vi "GEMV_Benchmark(lv_gpu).vi"() -> ()   [LabVIEW 2020]
doc: "Solves the heat equation in a two-dimensional area using a Finite Element Method."
uses:
  <vilib>/addons/lvgpu/lvcuda/CUDA SGL Device Ptr/Download 2D Data.vi
  <vilib>/addons/lvgpu/lvcublas/SGEMM (aAB+bC).vi
  <vilib>/addons/lvgpu/lvcuda/CUDA SGL Device Ptr/Upload 1D Data.vi
  <vilib>/addons/lvgpu/lvcuda.lvlib
  <vilib>/addons/lvgpu/lvcublas.lvlib
  subVIs/Heat Equation Solver.lvlib
  <vilib>/addons/lvgpu/lvcuda/CUDA SGL Device Ptr/CUDA SGL Device Ptr.lvclass
  <vilib>/ptbypt/NI_PtbyPt.lvlib
panel:
  out "Heat Map":sgl[](array[numeric])
  out "Execution Time Graph":dbl(graph)
  out "Error Status":errorcluster
  out "time":dbl[unit] format="%#_4p"
  in  "stop":bool
  # "GEMV based on NI's GPU Toolkit"
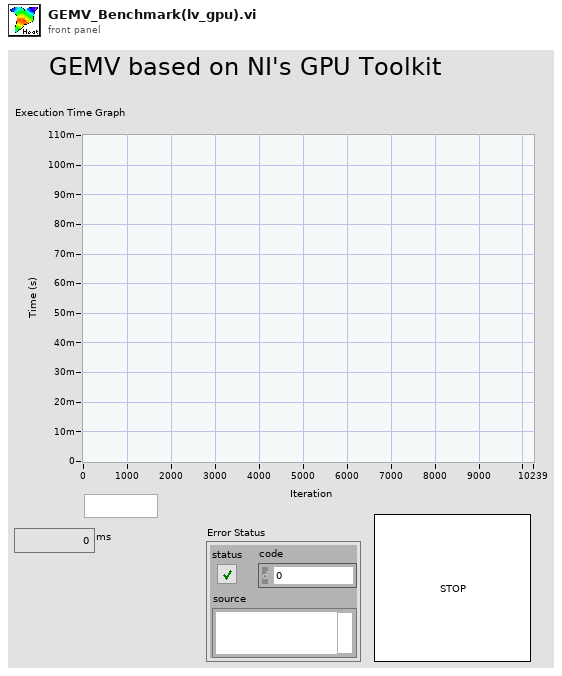
[diagram p1: front panel]
types:
  T1 = typedef "NI_Matrix.lvlib/RealMatrix.ctl" = dbl[][]
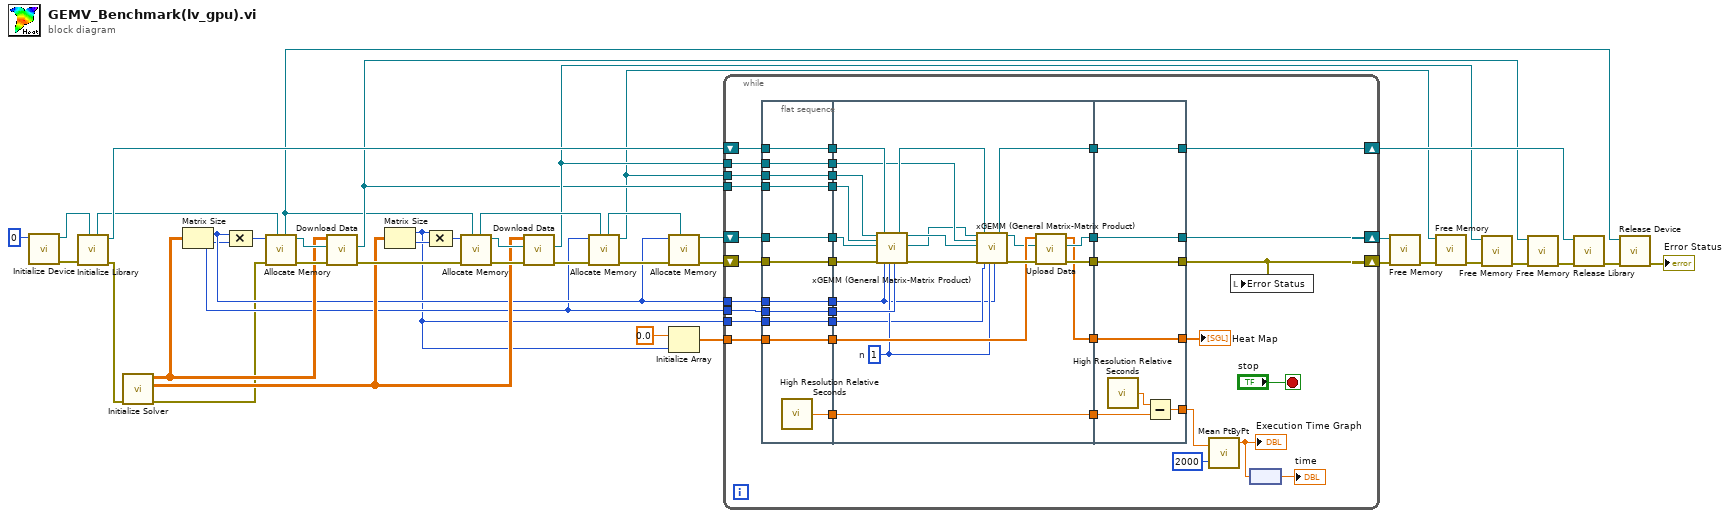
[diagram p0: block diagram]
diagram:
  n1 = call <vilib>:"Initialize Device.vi"("CUDA Device ID"=0 ("Device ID")) -> ("error out"=w39:errorcluster, "CUDA Context"=w40:refnum<class "CUDA Context.lvclass">)  [unwired: 8 in, 1 out]
  n2 = call <vilib>:"Initialize Library.vi"("CUDA Context in"=w40, "error in"=w39) -> ("error out"=w19:errorcluster, "CUBLAS Handle"=w41:refnum<class "CUBLAS Handle.lvclass">, "CUDA Context out"=w38:refnum<class "CUDA Context.lvclass">)  [unwired: 6 in, 1 out]
  n3 = call "Initialize Solver.vi"("error in"=w19) -> ("error out"=w2:errorcluster, "Mass"=w20:T1, "Stiffness"=w21:T1)  [unwired: 7 in, 1 out]
  n4 = Matrix Size(0:w21) -> (1:w6:i32, 2:w5:i32)
  n5 = Compound Arithmetic op=MULTIPLY(w6, w5) -> (w27:i32)
  n6 = call-poly <vilib>:"Allocate Memory.vi"("CUDA Context in"=w38, "error in"=w2, "size in elements"=w27) -> ("error out"=w25:errorcluster, "CUDA SGL Device Ptr out"=w35:refnum<class "CUDA SGL Device Ptr.lvclass">, "CUDA Context out"=w12:refnum<class "CUDA Context.lvclass">)  [unwired: 6 in]
  n7 = call-poly <vilib>:"Download Data.vi"("error in"=w25, "dst in"=w35, "src in"=w21) -> ("error out"=w24:errorcluster, "dst out"=w15:refnum<class "CUDA SGL Device Ptr.lvclass">)  [unwired: 6 in, 1 out]
  n8 = Matrix Size(0:w20) -> (1:w4:i32, 2:w26:i32)
  n9 = Compound Arithmetic op=MULTIPLY(w4, w26) -> (w36:i32)
  n10 = call-poly <vilib>:"Allocate Memory.vi"("CUDA Context in"=w12, "error in"=w24, "size in elements"=w36) -> ("error out"=w23:errorcluster, "CUDA SGL Device Ptr out"=w34:refnum<class "CUDA SGL Device Ptr.lvclass">, "CUDA Context out"=w37:refnum<class "CUDA Context.lvclass">)  [unwired: 6 in]
  n11 = call-poly <vilib>:"Download Data.vi"("error in"=w23, "dst in"=w34, "src in"=w20) -> ("error out"=w22:errorcluster, "dst out"=w16:refnum<class "CUDA SGL Device Ptr.lvclass">)  [unwired: 6 in, 1 out]
  n12 = call-poly <vilib>:"Allocate Memory.vi"("CUDA Context in"=w37, "error in"=w22, "size in elements"=w5) -> ("error out"=w11:errorcluster, "CUDA SGL Device Ptr out"=w8:refnum<class "CUDA SGL Device Ptr.lvclass">, "CUDA Context out"=w18:refnum<class "CUDA Context.lvclass">)  [unwired: 6 in]
  n13 = call-poly <vilib>:"Allocate Memory.vi"("CUDA Context in"=w18, "error in"=w11, "size in elements"=w6) -> ("error out"=w1:errorcluster, "CUDA SGL Device Ptr out"=w17:refnum<class "CUDA SGL Device Ptr.lvclass">)  [unwired: 6 in, 1 out]
  n14 = Initialize Array(sgl 0.0 ("SGL"), w4) -> (w9:sgl[])
  n15 = while {
    shift-right: [w53] -> w33
    shift-left: w41 -> [w66]
    shift-right: [w55] -> w14
    shift-left: w17 -> [w62]
    shift-right: [w54] -> w13
    shift-left: w1 -> [w60]
    tunnel: w16 -> [w70]
    tunnel: w15 -> [w69]
    tunnel: w8 -> [w64]
    tunnel: w6 -> [w50]
    tunnel: w9 -> [w58]
    tunnel: w5 -> [w48]
    tunnel: w4 -> [w46]
    stop <- "stop" stop-if-true
    n16 = flat-sequence {
      tunnel: w70 -> [w86]
      tunnel: w69 -> [w87]
      tunnel: [w87] -> w76
      tunnel: [w86] -> w75
      tunnel: [w85] -> w74
      tunnel: [w84] -> w67
      tunnel: w66 -> [w84]
      tunnel: [w83] -> w65
      tunnel: w64 -> [w83]
      tunnel: [w82] -> w63
      tunnel: w62 -> [w82]
      tunnel: [w81] -> w61
      tunnel: w60 -> [w81]
      tunnel: [w80] -> w59
      tunnel: w58 -> [w80]
      tunnel: [w79] -> w51
      tunnel: w50 -> [w79]
      tunnel: [w78] -> w49
      tunnel: w48 -> [w78]
      tunnel: [w77] -> w47
      tunnel: w46 -> [w77]
      tunnel: [w92] -> w73
      tunnel: w76 -> [w108]
      tunnel: w75 -> [w104]
      tunnel: w74 -> [w109]
      tunnel: [w109] -> w72
      tunnel: w67 -> [w107]
      tunnel: w65 -> [w102]
      tunnel: w63 -> [w103]
      tunnel: w61 -> [w101]
      tunnel: w59 -> [w97]
      tunnel: [w95] -> w57
      tunnel: [w94] -> w56
      tunnel: [w93] -> w52
      tunnel: w51 -> [w88]
      tunnel: w49 -> [w91]
      tunnel: w47 -> [w89]
      tunnel: [w116] -> w68
      tunnel: w73 -> [w116]
      tunnel: w72 -> [w115]
      tunnel: w57 -> [w112]
      tunnel: [w113] -> w55
      tunnel: w56 -> [w113]
      tunnel: [w112] -> w54
      tunnel: [w111] -> w53
      tunnel: w52 -> [w111]
      tunnel: [w110] -> w44
      frame #0 {
        n17 = call <vilib>:"High Resolution Relative Seconds.vi"() -> ("relative seconds"=w85:dbl)
      }
      frame #1 {
        w90 = 1  # n
        n18 = call-poly <vilib>:"xGEMM (General Matrix-Matrix Product).vi"("C"=w102, "A in"=w108, "B in"=w103, "error in"=w101, "CUBLAS Handle in"=w107, "m"=w88, "n"=w90, "k"=w91) -> ("CUBLAS Handle out"=w105:refnum<class "CUBLAS Handle.lvclass">, "aAB+bC"=w106:refnum<class "CUDA SGL Device Ptr.lvclass">, "B out"=w99:refnum<class "CUDA SGL Device Ptr.lvclass">, "error out"=w100:errorcluster)  [unwired: 7 in, 1 out]
        n19 = call-poly <vilib>:"xGEMM (General Matrix-Matrix Product).vi"("C"=w99, "A in"=w104, "B in"=w106, "error in"=w100, "CUBLAS Handle in"=w105, "m"=w89, "n"=w90, "k"=w88) -> ("CUBLAS Handle out"=w93:refnum<class "CUBLAS Handle.lvclass">, "aAB+bC"=w96:refnum<class "CUDA SGL Device Ptr.lvclass">, "error out"=w98:errorcluster)  [unwired: 7 in, 2 out]
        n20 = call-poly <vilib>:"Upload Data.vi"("error in"=w98, "src in"=w96, "dst in"=w97) -> ("error out"=w95:errorcluster, "src out"=w94:refnum<class "CUDA SGL Device Ptr.lvclass">, "dst out"=w92:sgl[])  [unwired: 6 in]
      }
      frame #2 {
        n21 = call <vilib>:"High Resolution Relative Seconds.vi"() -> ("relative seconds"=w114:dbl)
        n22 = Subtract(x=w114, y=w115) -> (x-y=w110:dbl)
      }
    }
    n23 = call <vilib>:"Mean PtByPt.vi"("x"=w44, "sample length"=2000) -> ("mean"=w43:dbl)  [unwired: 2 in, 1 out]
    "Execution Time Graph" <- w43
    n24 = local write "Error Status"(w54) -> ()
    n25 = node(w43) -> (→"time":dbl[unit])
    "Heat Map" <- w68
  }
  n26 = call-poly <vilib>:"Free Memory.vi"("error in"=w13, "CUDA SGL Device Ptr in"=w14) -> ("error out"=w28:errorcluster)  [unwired: 9 in]
  n27 = call-poly <vilib>:"Free Memory.vi"("error in"=w28, "CUDA SGL Device Ptr in"=w8) -> ("error out"=w29:errorcluster)  [unwired: 9 in]
  n28 = call-poly <vilib>:"Free Memory.vi"("error in"=w29, "CUDA SGL Device Ptr in"=w16) -> ("error out"=w30:errorcluster)  [unwired: 9 in]
  n29 = call-poly <vilib>:"Free Memory.vi"("error in"=w30, "CUDA SGL Device Ptr in"=w15) -> ("error out"=w31:errorcluster)  [unwired: 9 in]
  n30 = call <vilib>:"Release Library.vi"("error in"=w31, "CUBLAS Handle"=w33) -> ("error out"=w32:errorcluster)  [unwired: 9 in]
  n31 = call <vilib>:"Release Device.vi"("error in"=w32, "CUDA Context in"=w12) -> ("error out"=→"Error Status":errorcluster)  [unwired: 9 in]
